vi "Settings.vi"(8 "Error In":errorcluster, 10 "Manual":path=path "", 11 "Settings in":T11={"MFIA"={"Address"="", "Use compensation"=TRUE, "Shut down gracefully"=FALSE}, "Temp ctrl"={"Gain (P)"=0.0, "Reset (I)"=0.0, "Rate (D)"=0.0, "Stabilization rate"=0.0, "Stabilization delta"=0.0, "Type"=enum."Lake Shore 325", "Custom temp ctrl"={"VISA resource name"=""}, "Lakeshore 325"={"VISA name"="", "Loop"=0, "Heater Range"=1, "Heater Resistance"=0, "Sample sensor"=0, "Fast sensor"=0, "Slow sensor"=0}, "Lakeshore 331"={"VISA name"="", "Loop"=1, "Heater Range"=0, "Sample sensor"=0, "Fast sensor"=0, "Slow sensor"=0}, "Lakeshore 332"={"VISA name"="", "Loop"=1, "Heater Range"=0, "Sample sensor"=0, "Fast sensor"=0, "Slow sensor"=0}, "Lakeshore 335"={"VISA name"="", "Loop"=1, "Sample sensor"=0, "Fast sensor"=0, "Slow sensor"=0, "Heater Range"=0, "Heater Output"=1, "Output mode"=enum."Off"}}, "Source-meter"={"Type"=enum."Custom", "Custom source-meter"={"VISA resource name"=""}, "Keithley 2600"={"VISA name"=""}}, "Other"={"Enable OriginLab"=FALSE, "Reader mode"=FALSE, "Auto-save"=FALSE}, "Defaults"={"IV properties"={"T"=0.0, "Vstart"=-0.5, "Vstop"=0.5, "Vpoints"=10.0, "Settling"=0.01, "I limit"=-3.0, "Log mapping"=FALSE, "Averaging"=0.0}, "CV properties"={"T"=0.0, "Vstart"=-0.5, "Vstop"=0.5, "Vpoints"=10.0, "Precision"=enum."Normal", "Test signal"=0.01, "Auto I range"=FALSE, "Test frequency"=100000.0, "I range"=-2.0, "V range"=10.0, "Log mapping"=FALSE, "Rel perm"=0.0, "Area"=0.0}, "DLTS properties"={"Tstart"=0.0, "Instant start"=FALSE, "Tstop"=0.0, "T rate"=0.0, "Test signal"=0.0, "Test frequency"=0.0, "Bandwidth"=0.0, "Averaging"=0.0, "Vbias"=0.0, "Vpulse"=0.0, "pulse length"=0.0, "Pulse 2"=FALSE, "Vpulse 2"=0.0, "pulse length 2"=0.0, "I range"=-2.0, "V range"=10.0, "Emission rate"=[], "Sampling rate"=0.0, "Acq. delay"=0.0}, "LDLTS properties"={"T"=0.0, "Test signal"=0.0, "Test frequency"=0.0, "Bandwidth"=0.0, "Averaging"=0.0, "Vbias"=0.0, "Vpulse"=0.0, "pulse length"=0.0, "Pulse 2"=FALSE, "Vpulse 2"=0.0, "pulse length 2"=0.0, "I range"=-2.0, "V range"=10.0, "Sampling rate"=0.0, "Acq. delay"=0.0, "Sampling time"=0.0}}} {"Defaults"."LDLTS properties"."V range" items=["10mV"=0.01, "100mV"=0.1, "1V"=1.0, "10V"=10.0]; "Defaults"."LDLTS properties"."I range" items=["100nA"=-7.0, "1µA"=-6.0, "10µA"=-5.0, "100µA"=-4.0, "1mA"=-3.0, "10mA"=-2.0]; "Defaults"."DLTS properties"."V range" items=["10mV"=0.01, "100mV"=0.1, "1V"=1.0, "10V"=10.0]; "Defaults"."DLTS properties"."I range" items=["10mV"=0.01, "100mV"=0.1, "1V"=1.0, "10V"=10.0]; "Defaults"."CV properties"."V range" items=["10mV"=0.01, "100mV"=0.1, "1V"=1.0, "10V"=10.0]; "Defaults"."CV properties"."I range" items=["100nA"=-7.0, "1µA"=-6.0, "10µA"=-5.0, "100µA"=-4.0, "1mA"=-3.0, "10mA"=-2.0]; "Defaults"."IV properties"."Settling" min=0.0 max=65535.0; "Temp ctrl"."Lakeshore 335"."Heater Output" items=["1"=1, "2"=2]; "Temp ctrl"."Lakeshore 335"."Heater Range" items=["Off", "Low (On)", "Medium", "High"]; "Temp ctrl"."Lakeshore 335"."Slow sensor" items=["A", "B"]; "Temp ctrl"."Lakeshore 335"."Fast sensor" items=["A", "B"]; "Temp ctrl"."Lakeshore 335"."Sample sensor" items=["A", "B"]; "Temp ctrl"."Lakeshore 335"."Loop" items=["Loop 1"=1, "Loop 2"=2]; "Temp ctrl"."Lakeshore 332"."Slow sensor" items=["A", "B"]; "Temp ctrl"."Lakeshore 332"."Fast sensor" items=["A", "B"]; "Temp ctrl"."Lakeshore 332"."Sample sensor" items=["A", "B"]; "Temp ctrl"."Lakeshore 332"."Heater Range" items=["Off", "Low (0.5W)", "Med (5W)", "High (50W)"]; "Temp ctrl"."Lakeshore 332"."Loop" items=["Loop 1", "Loop 2"]; "Temp ctrl"."Lakeshore 331"."Slow sensor" items=["A", "B"]; "Temp ctrl"."Lakeshore 331"."Fast sensor" items=["A", "B"]; "Temp ctrl"."Lakeshore 331"."Sample sensor" items=["A", "B"]; "Temp ctrl"."Lakeshore 331"."Heater Range" items=["Off", "Low (0.5W)", "Med (5W)", "High (50W)"]; "Temp ctrl"."Lakeshore 331"."Loop" items=["Loop 1", "Loop 2"]; "Temp ctrl"."Lakeshore 325"."Slow sensor" items=["A", "B"]; "Temp ctrl"."Lakeshore 325"."Fast sensor" items=["A", "B"]; "Temp ctrl"."Lakeshore 325"."Sample sensor" items=["A", "B"]; "Temp ctrl"."Lakeshore 325"."Heater Resistance" items=["25 Ohm"=1, "50 Ohm"=2]; "Temp ctrl"."Lakeshore 325"."Heater Range" items=["Off", "Low (loop 1) or On (loop 2)", "High (loop 1)"]; "Temp ctrl"."Lakeshore 325"."Loop" items=["Loop 1"=1, "Loop 2"=2]}) -> (0 "Error Out":errorcluster, 3 "Settings":T11={"MFIA"={"Address"="", "Use compensation"=TRUE, "Shut down gracefully"=FALSE}, "Temp ctrl"={"Gain (P)"=0.0, "Reset (I)"=0.0, "Rate (D)"=0.0, "Stabilization rate"=0.0, "Stabilization delta"=0.0, "Type"=enum."Lake Shore 325", "Custom temp ctrl"={"VISA resource name"=""}, "Lakeshore 325"={"VISA name"="", "Loop"=0, "Heater Range"=1, "Heater Resistance"=0, "Sample sensor"=0, "Fast sensor"=0, "Slow sensor"=0}, "Lakeshore 331"={"VISA name"="", "Loop"=1, "Heater Range"=0, "Sample sensor"=0, "Fast sensor"=0, "Slow sensor"=0}, "Lakeshore 332"={"VISA name"="", "Loop"=1, "Heater Range"=0, "Sample sensor"=0, "Fast sensor"=0, "Slow sensor"=0}, "Lakeshore 335"={"VISA name"="", "Loop"=1, "Sample sensor"=0, "Fast sensor"=0, "Slow sensor"=0, "Heater Range"=0, "Heater Output"=1, "Output mode"=enum."Off"}}, "Source-meter"={"Type"=enum."Custom", "Custom source-meter"={"VISA resource name"=""}, "Keithley 2600"={"VISA name"=""}}, "Other"={"Enable OriginLab"=FALSE, "Reader mode"=FALSE, "Auto-save"=FALSE}, "Defaults"={"IV properties"={"T"=0.0, "Vstart"=-0.5, "Vstop"=0.5, "Vpoints"=10.0, "Settling"=0.01, "I limit"=-3.0, "Log mapping"=FALSE, "Averaging"=0.0}, "CV properties"={"T"=0.0, "Vstart"=-0.5, "Vstop"=0.5, "Vpoints"=10.0, "Precision"=enum."Normal", "Test signal"=0.01, "Auto I range"=FALSE, "Test frequency"=100000.0, "I range"=-2.0, "V range"=10.0, "Log mapping"=FALSE, "Rel perm"=0.0, "Area"=0.0}, "DLTS properties"={"Tstart"=0.0, "Instant start"=FALSE, "Tstop"=0.0, "T rate"=0.0, "Test signal"=0.0, "Test frequency"=0.0, "Bandwidth"=0.0, "Averaging"=0.0, "Vbias"=0.0, "Vpulse"=0.0, "pulse length"=0.0, "Pulse 2"=FALSE, "Vpulse 2"=0.0, "pulse length 2"=0.0, "I range"=-2.0, "V range"=10.0, "Emission rate"=[], "Sampling rate"=0.0, "Acq. delay"=0.0}, "LDLTS properties"={"T"=0.0, "Test signal"=0.0, "Test frequency"=0.0, "Bandwidth"=0.0, "Averaging"=0.0, "Vbias"=0.0, "Vpulse"=0.0, "pulse length"=0.0, "Pulse 2"=FALSE, "Vpulse 2"=0.0, "pulse length 2"=0.0, "I range"=-2.0, "V range"=10.0, "Sampling rate"=0.0, "Acq. delay"=0.0, "Sampling time"=0.0}}} {"Defaults"."LDLTS properties"."V range" items=["10mV"=0.01, "100mV"=0.1, "1V"=1.0, "10V"=10.0]; "Defaults"."LDLTS properties"."I range" items=["100nA"=-7.0, "1µA"=-6.0, "10µA"=-5.0, "100µA"=-4.0, "1mA"=-3.0, "10mA"=-2.0]; "Defaults"."DLTS properties"."V range" items=["10mV"=0.01, "100mV"=0.1, "1V"=1.0, "10V"=10.0]; "Defaults"."DLTS properties"."I range" items=["10mV"=0.01, "100mV"=0.1, "1V"=1.0, "10V"=10.0]; "Defaults"."CV properties"."V range" items=["10mV"=0.01, "100mV"=0.1, "1V"=1.0, "10V"=10.0]; "Defaults"."CV properties"."I range" items=["100nA"=-7.0, "1µA"=-6.0, "10µA"=-5.0, "100µA"=-4.0, "1mA"=-3.0, "10mA"=-2.0]; "Defaults"."IV properties"."Settling" min=0.0 max=65535.0; "Temp ctrl"."Lakeshore 335"."Heater Output" items=["1"=1, "2"=2]; "Temp ctrl"."Lakeshore 335"."Heater Range" items=["Off", "Low (On)", "Medium", "High"]; "Temp ctrl"."Lakeshore 335"."Slow sensor" items=["A", "B"]; "Temp ctrl"."Lakeshore 335"."Fast sensor" items=["A", "B"]; "Temp ctrl"."Lakeshore 335"."Sample sensor" items=["A", "B"]; "Temp ctrl"."Lakeshore 335"."Loop" items=["Loop 1"=1, "Loop 2"=2]; "Temp ctrl"."Lakeshore 332"."Slow sensor" items=["A", "B"]; "Temp ctrl"."Lakeshore 332"."Fast sensor" items=["A", "B"]; "Temp ctrl"."Lakeshore 332"."Sample sensor" items=["A", "B"]; "Temp ctrl"."Lakeshore 332"."Heater Range" items=["Off", "Low (0.5W)", "Med (5W)", "High (50W)"]; "Temp ctrl"."Lakeshore 332"."Loop" items=["Loop 1", "Loop 2"]; "Temp ctrl"."Lakeshore 331"."Slow sensor" items=["A", "B"]; "Temp ctrl"."Lakeshore 331"."Fast sensor" items=["A", "B"]; "Temp ctrl"."Lakeshore 331"."Sample sensor" items=["A", "B"]; "Temp ctrl"."Lakeshore 331"."Heater Range" items=["Off", "Low (0.5W)", "Med (5W)", "High (50W)"]; "Temp ctrl"."Lakeshore 331"."Loop" items=["Loop 1", "Loop 2"]; "Temp ctrl"."Lakeshore 325"."Slow sensor" items=["A", "B"]; "Temp ctrl"."Lakeshore 325"."Fast sensor" items=["A", "B"]; "Temp ctrl"."Lakeshore 325"."Sample sensor" items=["A", "B"]; "Temp ctrl"."Lakeshore 325"."Heater Resistance" items=["25 Ohm"=1, "50 Ohm"=2]; "Temp ctrl"."Lakeshore 325"."Heater Range" items=["Off", "Low (loop 1) or On (loop 2)", "High (loop 1)"]; "Temp ctrl"."Lakeshore 325"."Loop" items=["Loop 1"=1, "Loop 2"=2]})   [LabVIEW 2019]
doc: "Displays a window that enabling user to modify the settings"
uses:
  Type defs/Settings Type Def.ctl
  Type defs/Imps Type Def.ctl
  Type defs/Temp ctrl Type Def.ctl
  Custom devices/Custom temp ctrl settings.ctl
  Type defs/Source-meter Type Def.ctl
  Custom devices/Custom source-meter settings.ctl
  Type defs/Other settings Type Def.ctl
  Type defs/IV properties Type Def.ctl
  Type defs/CV properties Type Def.ctl
  Type defs/DLTS properties Type Def.ctl
  Type defs/LDLTS properties Type Def.ctl
  <vilib>/Utility/miscctls.llb/LVPointTypeDef.ctl
  <instrlib>/Zurich Instruments LabOne/Zurich Instruments LabOne.lvlib
panel:
  in  "Help":bool
  in  "Tab Control":T1(tab)
  in  "Address":string(combo) caption="Combo Box"
  in  "Refresh":bool
  in  "Use user compensation":bool
  in  "Safely shutdown on exit":bool
  in  "Stabilization delta":dbl[unit] caption="Numeric"
  in  "Stabilization rate":dbl[unit] caption="Numeric"
  in  "Temp type":T2(tab)
  in  "Custom temp ctrl":T3
  in  "Fast sensor LS325":u16(ring)=1 caption="Fast sensor" items=["Sensor A", "Sensor B"]
  in  "Slow sensor LS325":u16(ring)=1 caption="Slow sensor" items=["Sensor A", "Sensor B"]
  in  "Sample sensor LS325":u16(ring)=1 caption="Sample sensor" items=["Sensor A", "Sensor B"]
  in  "Heater range LS325":u16(ring)=1 caption="Heater range" items=["Off", "Low (L1)/On (L2)", "High (L1)"]
  in  "Loop  LS325":u16(ring)=1 caption="Loop" items=["Loop 1"=1, "Loop 2"=2]
  in  "VISA name LS325":refnum<visa-resource-name> caption="VISA name"
  in  "Heater resistance LS325":u16(ring)=1 caption="Heater resistance" items=["25 Ohm"=1, "50 Ohm"=2]
  in  "Fast sensor LS331":u16(ring)=1 caption="Fast sensor" items=["Sensor A", "Sensor B"]
  in  "Slow sensor LS331":u16(ring)=1 caption="Slow sensor" items=["Sensor A", "Sensor B"]
  in  "Sample sensor LS331":u16(ring)=1 caption="Sample sensor" items=["Sensor A", "Sensor B"]
  in  "Heater range LS331":u16(ring)=1 caption="Heater range" items=["Off", "Low (0.5W)", "Med (5W)", "High (50W)"]
  in  "Loop  LS331":u16(ring)=1 caption="Loop" items=["Loop 1", "Loop 2"]
  in  "VISA name LS331":refnum<visa-resource-name> caption="VISA name"
  in  "Fast sensor LS332":u16(ring)=1 caption="Fast sensor" items=["Sensor A", "Sensor B"]
  in  "Slow sensor LS332":u16(ring)=1 caption="Slow sensor" items=["Sensor A", "Sensor B"]
  in  "Sample sensor LS332":u16(ring)=1 caption="Sample sensor" items=["Sensor A", "Sensor B"]
  in  "Heater range LS332":u16(ring)=1 caption="Heater range" items=["Off", "Low (0.5W)", "Med (5W)", "High (50W)"]
  in  "Loop  LS332":u16(ring)=1 caption="Loop" items=["Loop 1", "Loop 2"]
  in  "VISA name LS332":refnum<visa-resource-name> caption="VISA name"
  in  "Heater range LS335":enum16{"Off", "Low/On", "Medium", "High"}(ring) caption="Heater range"
  in  "Output mode LS335":T4(ring) caption="Output mode"
  in  "Heater output LS335":u16=1 caption="Heater output" min=1 max=2 step=1
  in  "Fast sensor LS335":u16(ring)=1 caption="Fast sensor" items=["Sensor A", "Sensor B"]
  in  "Slow sensor LS335":u16(ring)=1 caption="Slow sensor" items=["Sensor A", "Sensor B"]
  in  "Sample sensor LS335":u16(ring)=1 caption="Sample sensor" items=["Sensor A", "Sensor B"]
  in  "Loop  LS335":u16(ring)=1 caption="Loop" items=["Loop 1"=1, "Loop 2"=2]
  in  "VISA name LS335":refnum<visa-resource-name> caption="VISA name"
  in  "PID":T5
  in  "Source-meter type":enum32{"Custom", "Keithley 2600"}(tab)
  in  "Custom source-meter":T6
  in  "VISA name Keithley 2600":refnum<visa-resource-name> caption="VISA name"
  in  "Defaults tab control":enum32{"CV", "IV", "DLTS", "LDLTS"}(tab)
  in  "CV properties":T7={"T"=0.0, "Vstart"=-0.5, "Vstop"=0.5, "Vpoints"=10.0, "Precision"=enum."Normal", "Test signal"=0.01, "Auto I range"=FALSE, "Test frequency"=100000.0, "I range"=-2.0, "V range"=10.0, "Log mapping"=FALSE, "Rel perm"=0.0, "Area"=0.0} {"V range" items=["10mV"=0.01, "100mV"=0.1, "1V"=1.0, "10V"=10.0]; "I range" items=["100nA"=-7.0, "1µA"=-6.0, "10µA"=-5.0, "100µA"=-4.0, "1mA"=-3.0, "10mA"=-2.0]}
  in  "IV properties":T8={"T"=0.0, "Vstart"=-0.5, "Vstop"=0.5, "Vpoints"=10.0, "Settling"=0.01, "I limit"=-3.0, "Log mapping"=FALSE, "Averaging"=0.0} {"Settling" min=0.0 max=65535.0}
  in  "DLTS properties":T9={"Tstart"=0.0, "Instant start"=FALSE, "Tstop"=0.0, "T rate"=0.0, "Test signal"=0.0, "Test frequency"=0.0, "Bandwidth"=0.0, "Averaging"=0.0, "Vbias"=0.0, "Vpulse"=0.0, "pulse length"=0.0, "Pulse 2"=FALSE, "Vpulse 2"=0.0, "pulse length 2"=0.0, "I range"=-2.0, "V range"=10.0, "Emission rate"=[], "Sampling rate"=0.0, "Acq. delay"=0.0} {"Sampling rate" items=["13k"=13392.857422, "27k"=26785.714844, "54k"=53571.429687, "107k"=107142.859375]; "V range" items=["10mV"=0.01, "100mV"=0.1, "1V"=1.0, "10V"=10.0]; "I range" items=["100nA"=-7.0, "1µA"=-6.0, "10µA"=-5.0, "100µA"=-4.0, "1mA"=-3.0, "10mA"=-2.0]}
  in  "LDLTS properties":T10={"T"=0.0, "Test signal"=0.0, "Test frequency"=0.0, "Bandwidth"=0.0, "Averaging"=0.0, "Vbias"=0.0, "Vpulse"=0.0, "pulse length"=0.0, "Pulse 2"=FALSE, "Vpulse 2"=0.0, "pulse length 2"=0.0, "I range"=-2.0, "V range"=10.0, "Sampling rate"=0.0, "Acq. delay"=0.0, "Sampling time"=0.0} {"Sampling rate" items=["13k"=13392.857422, "27k"=26785.714844, "54k"=53571.429687, "107k"=107142.859375]; "V range" items=["10mV"=0.01, "100mV"=0.1, "1V"=1.0, "10V"=10.0]; "I range" items=["100nA"=-7.0, "1µA"=-6.0, "10µA"=-5.0, "100µA"=-4.0, "1mA"=-3.0, "10mA"=-2.0]}
  in  "Reader mode":bool
  in  "Enable Origin":bool caption="Enable OriginLab"
  in  "Auto-save":bool
  in  "Cancel":bool
  in  "Apply All":bool
  # "Warning! This device has not been tested with myDLTS"
  # "Warning! This device has not been tested with myDLTS"
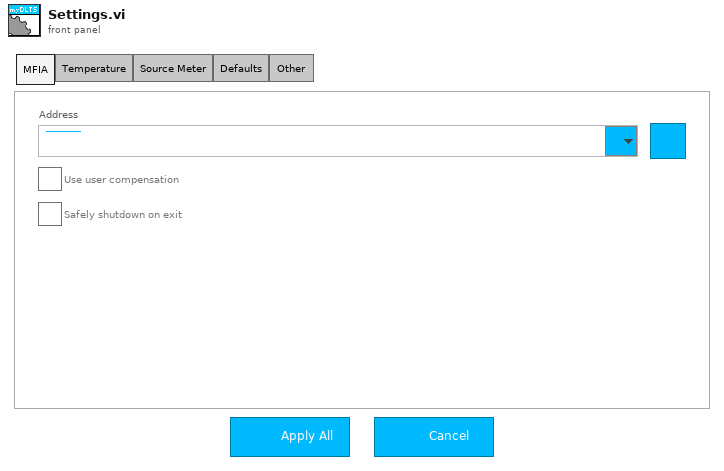
[diagram p1: front panel]
types:
  T1 = enum32{"MFIA", "Temperature", "Source Meter", "Defaults", "Other "}
  T2 = enum32{"Custom", "Lake Shore 325", "Lake Shore 331", "Lake Shore 332", "Lake Shore 335"}
  T3 = typedef "Custom temp ctrl settings.ctl" = cluster{"VISA resource name":refnum<visa-resource-name>}
  T4 = enum16{"Off", "Closed Loop PID", "Zone", "Open Loop", "Monitor Out", "Warmup Supply"}
  T5 = cluster{"Gain (P)":dbl, "Reset (I)":dbl, "Rate (D)":u16}
  T6 = typedef "Custom source-meter settings.ctl" = cluster{"VISA resource name":refnum<visa-resource-name>}
  T7 = typedef "CV properties Type Def.ctl" = cluster{"T":dbl[unit], "Vstart":dbl[unit], "Vstop":dbl[unit], "Vpoints":dbl, "Precision":enum16{"Low (Fast)", "Normal", "High (Slow)"}, "Test signal":dbl[unit], "Auto I range":bool, "Test frequency":dbl[unit], "I range":dbl, "V range":dbl[unit], "Log mapping":bool, "Rel perm":dbl, "Area":dbl[unit]}
  T8 = typedef "IV properties Type Def.ctl" = cluster{"T":dbl[unit], "Vstart":dbl[unit], "Vstop":dbl[unit], "Vpoints":dbl, "Settling":dbl[unit], "I limit":dbl[unit], "Log mapping":bool, "Averaging":dbl}
  T9 = typedef "DLTS properties Type Def.ctl" = cluster{"Tstart":dbl[unit], "Instant start":bool, "Tstop":dbl[unit], "T rate":dbl[unit], "Test signal":dbl[unit], "Test frequency":dbl[unit], "Bandwidth":dbl[unit], "Averaging":dbl, "Vbias":dbl[unit], "Vpulse":dbl[unit], "pulse length":dbl[unit], "Pulse 2":bool, "Vpulse 2":dbl[unit], "pulse length 2":dbl[unit], "I range":dbl, "V range":dbl[unit], "Emission rate":dbl[unit][], "Sampling rate":dbl[unit], "Acq. delay":dbl[unit]}
  T10 = typedef "LDLTS properties Type Def.ctl" = cluster{"T":dbl[unit], "Test signal":dbl[unit], "Test frequency":dbl[unit], "Bandwidth":dbl[unit], "Averaging":dbl, "Vbias":dbl[unit], "Vpulse":dbl[unit], "pulse length":dbl[unit], "Pulse 2":bool, "Vpulse 2":dbl[unit], "pulse length 2":dbl[unit], "I range":dbl, "V range":dbl[unit], "Sampling rate":dbl[unit], "Acq. delay":dbl[unit], "Sampling time":dbl[unit]}
  T11 = typedef "Settings Type Def.ctl" = cluster{"MFIA":T12, "Temp ctrl":T13, "Source-meter":T14, "Other":T15, "Defaults":cluster{"IV properties":T8, "CV properties":T7, "DLTS properties":T9, "LDLTS properties":T10}}
  T12 = typedef "Imps Type Def.ctl" = cluster{"Address":string, "Use compensation":bool, "Shut down gracefully":bool}
  T13 = typedef "Temp ctrl Type Def.ctl" = cluster{"Gain (P)":dbl, "Reset (I)":dbl, "Rate (D)":dbl, "Stabilization rate":dbl, "Stabilization delta":dbl, "Type":enum16{"Custom", "Lake Shore 325", "Lake Shore 331", "Lake Shore 332", "Lake Shore 335"}, "Custom temp ctrl":T3, "Lakeshore 325":cluster{"VISA name":refnum<visa-resource-name>, "Loop":u16, "Heater Range":u16, "Heater Resistance":u16, "Sample sensor":u16, "Fast sensor":u16, "Slow sensor":u16}, "Lakeshore 331":cluster{"VISA name":refnum<visa-resource-name>, "Loop":u16, "Heater Range":u16, "Sample sensor":u16, "Fast sensor":u16, "Slow sensor":u16}, "Lakeshore 332":cluster{"VISA name":refnum<visa-resource-name>, "Loop":u16, "Heater Range":u16, "Sample sensor":u16, "Fast sensor":u16, "Slow sensor":u16}, "Lakeshore 335":cluster{"VISA name":refnum<visa-resource-name>, "Loop":u16, "Sample sensor":u16, "Fast sensor":u16, "Slow sensor":u16, "Heater Range":u16, "Heater Output":u16, "Output mode":enum16{"Off", "Closed Loop PID", "Zone", "Open Loop", "Monitor Out", "Warmup Supply"}}}
  T14 = typedef "Source-meter Type Def.ctl" = cluster{"Type":enum16{"Custom", "Keithley 2600"}, "Custom source-meter":T6, "Keithley 2600":cluster{"VISA name":refnum<visa-resource-name>}}
  T15 = typedef "Other settings Type Def.ctl" = cluster{"Enable OriginLab":bool, "Reader mode":bool, "Auto-save":bool}
  T16 = typedef "LVPointTypeDef.ctl" = cluster{"Horizontal":i16, "Vertical":i16}
  T17 = enum16{"Custom", "Lake Shore 325", "Lake Shore 331", "Lake Shore 332", "Lake Shore 335"}
  T18 = cluster{"Rate (D)":dbl, "Reset (I)":dbl, "Gain (P)":dbl}
  T19 = enum8{"Enabled", "Disabled", "Disabled and Grayed Out"}
  T20 = cluster{"VISA name LS335":refnum<visa-resource-name>, "Loop  LS335":u16, "Sample sensor LS335":u16, "Fast sensor LS335":u16, "Slow sensor LS335":u16, "Heater range LS335":enum16{"Off", "Low/On", "Medium", "High"}, "Heater output LS335":u16, "Output mode LS335":enum16{"Off", "Closed Loop PID", "Zone", "Open Loop", "Monitor Out", "Warmup Supply"}}
  T21 = cluster{"VISA name LS332":refnum<visa-resource-name>, "Loop  LS332":u16, "Heater range LS332":u16, "Sample sensor LS332":u16, "Fast sensor LS332":u16, "Slow sensor LS332":u16}
  T22 = cluster{"VISA name LS331":refnum<visa-resource-name>, "Loop  LS331":u16, "Heater range LS331":u16, "Sample sensor LS331":u16, "Fast sensor LS331":u16, "Slow sensor LS331":u16}
  T23 = typedef "Zurich Instruments LabOne.lvlib/ziTypeHandle.ctl" = cluster{"handleValid":bool, "Conn":u64, "Path Prefix":string, "Handle":u64, "Connected":bool, "Clockbase(s)":dbl}
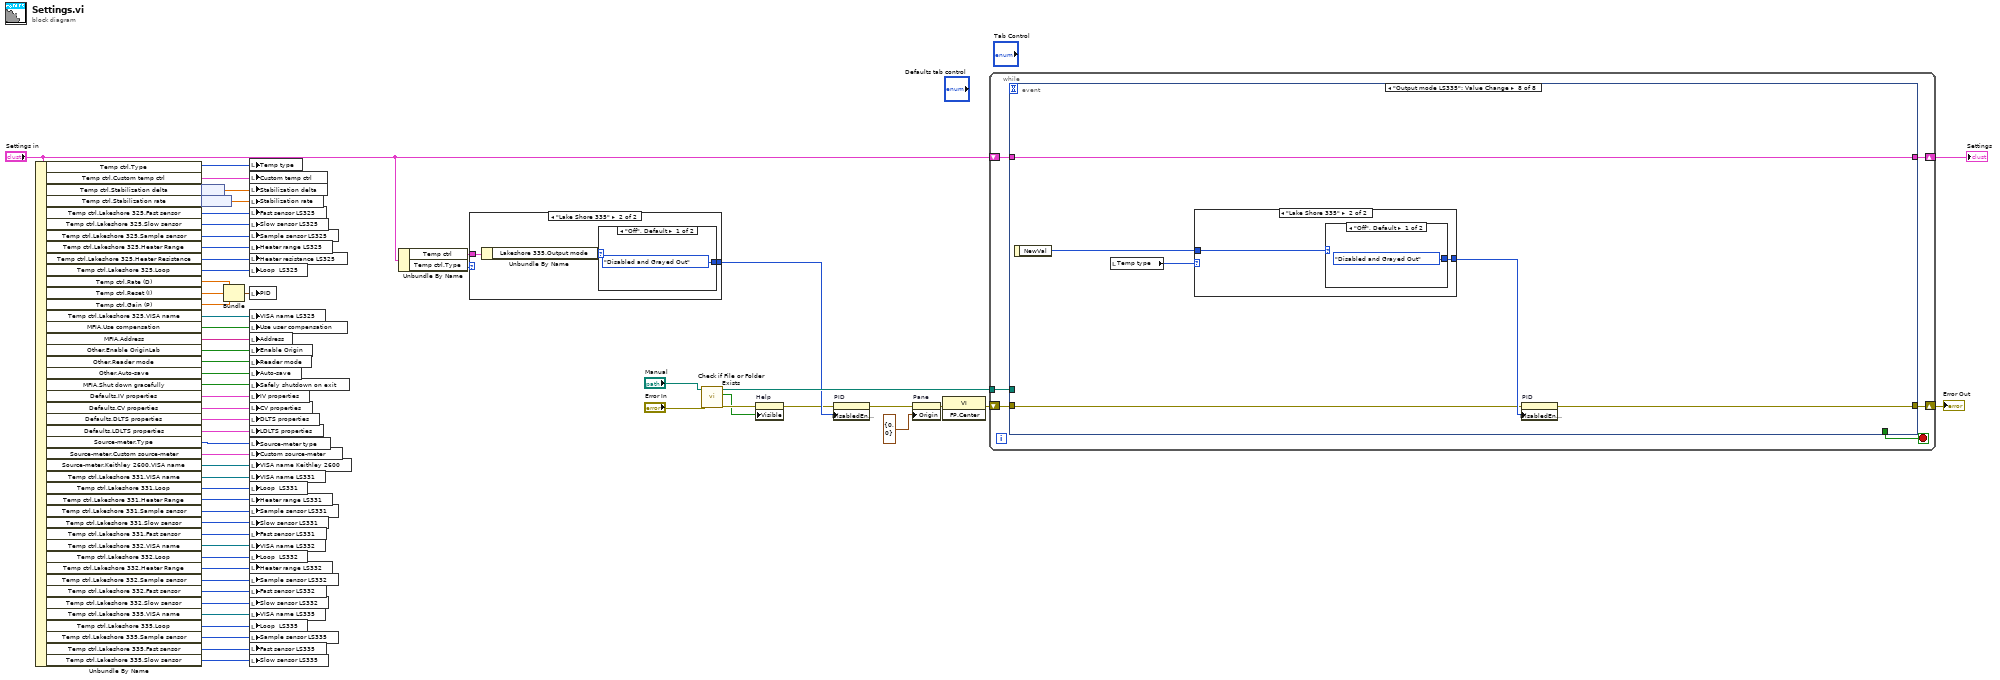
[diagram p0: block diagram]
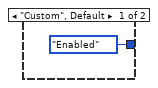
[diagram p2: hidden frame]
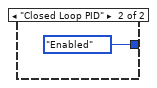
[diagram p3: hidden frame]
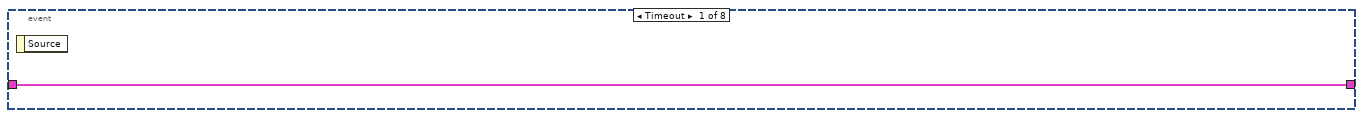
[diagram p4: hidden frame]
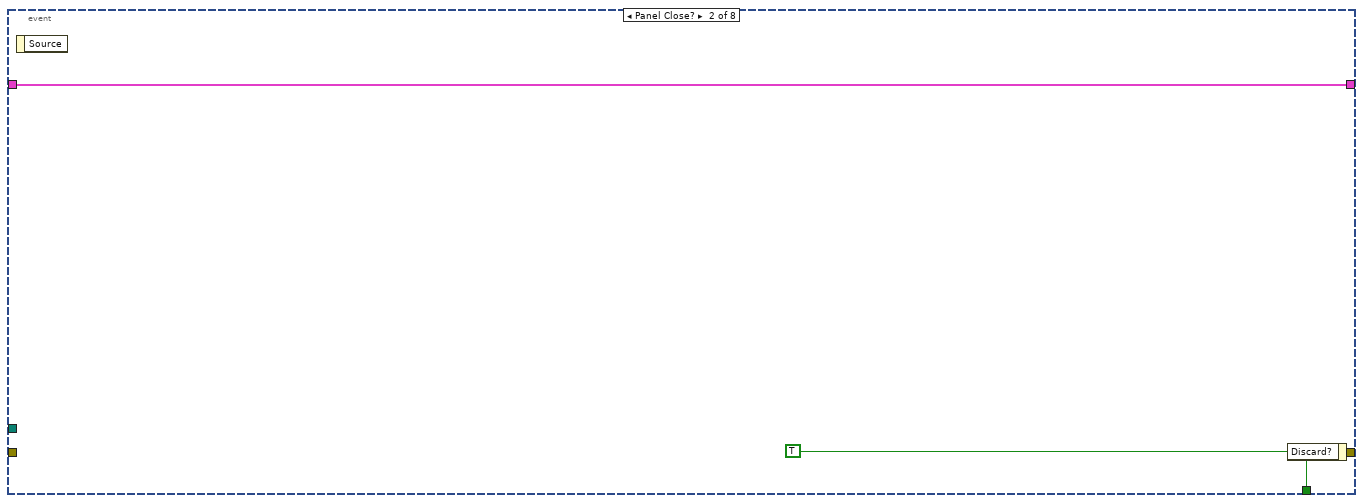
[diagram p5: hidden frame]
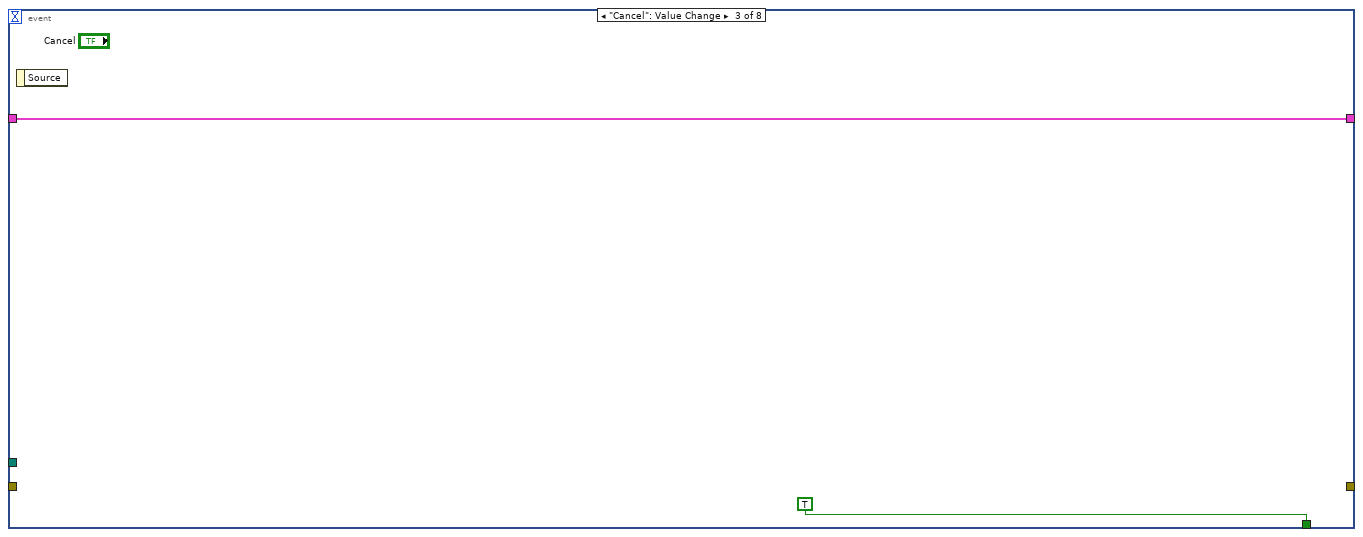
[diagram p6: hidden frame]
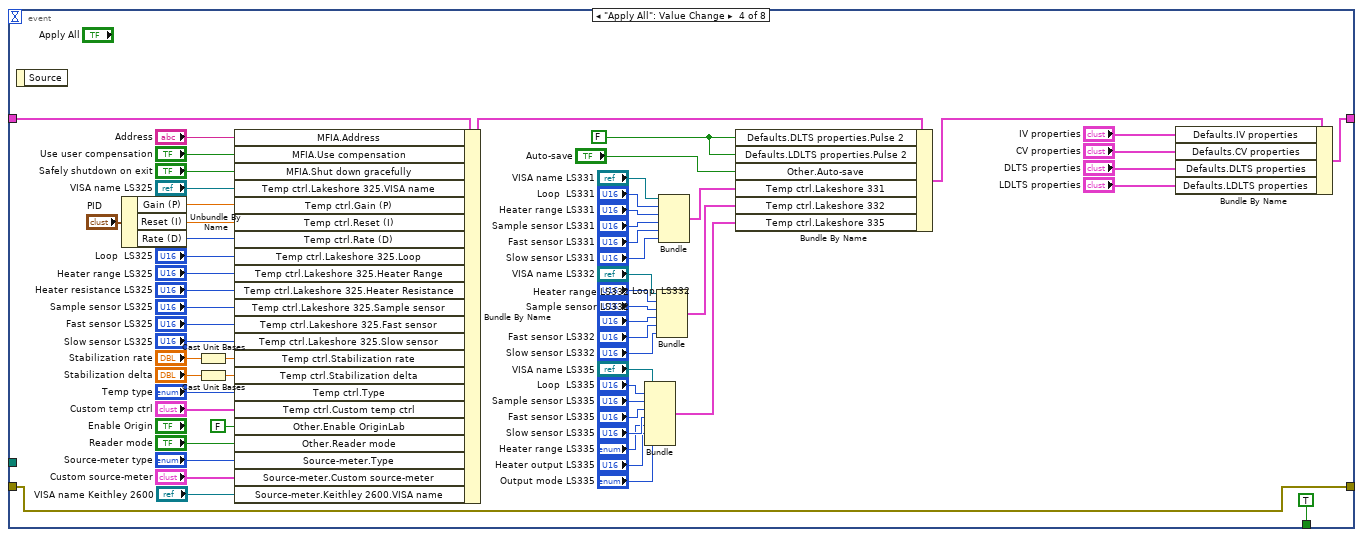
[diagram p7: hidden frame]
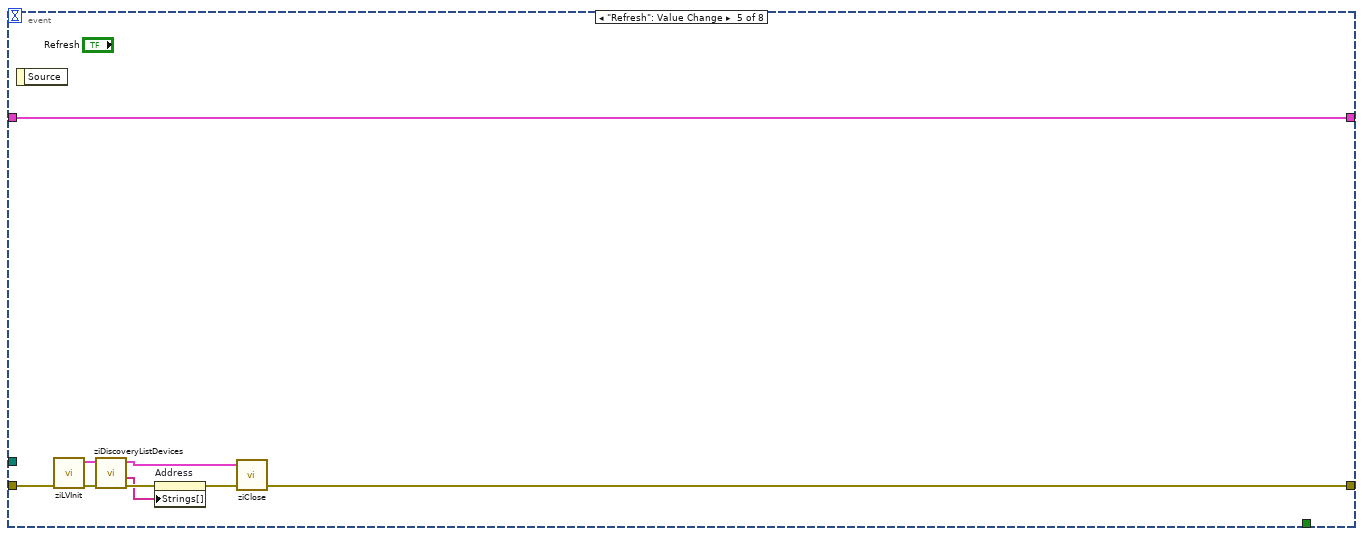
[diagram p8: hidden frame]
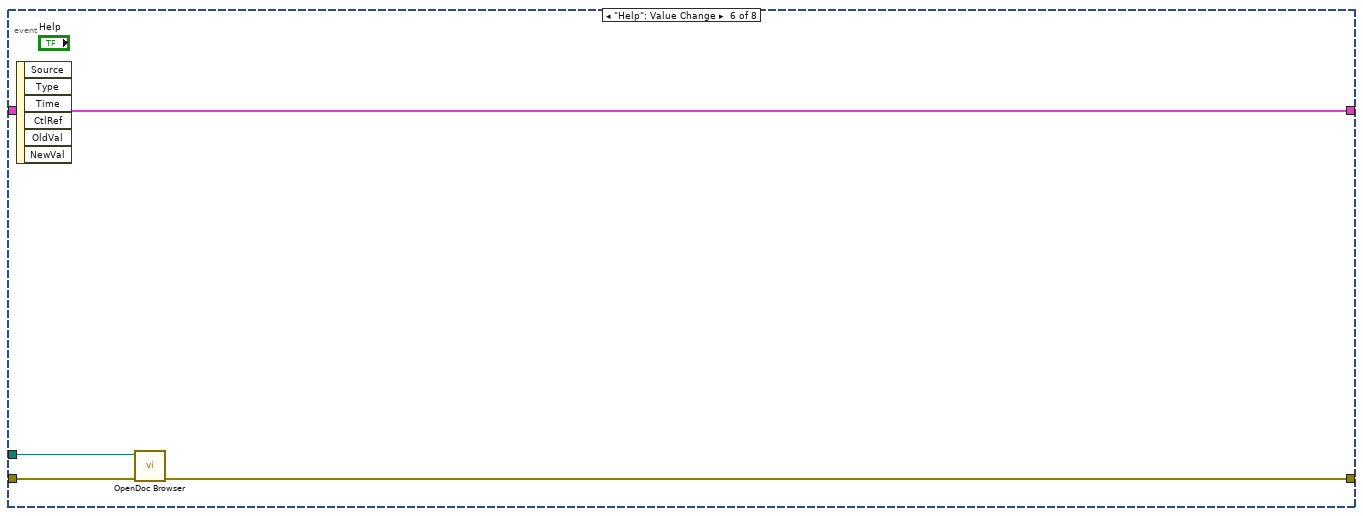
[diagram p9: hidden frame]
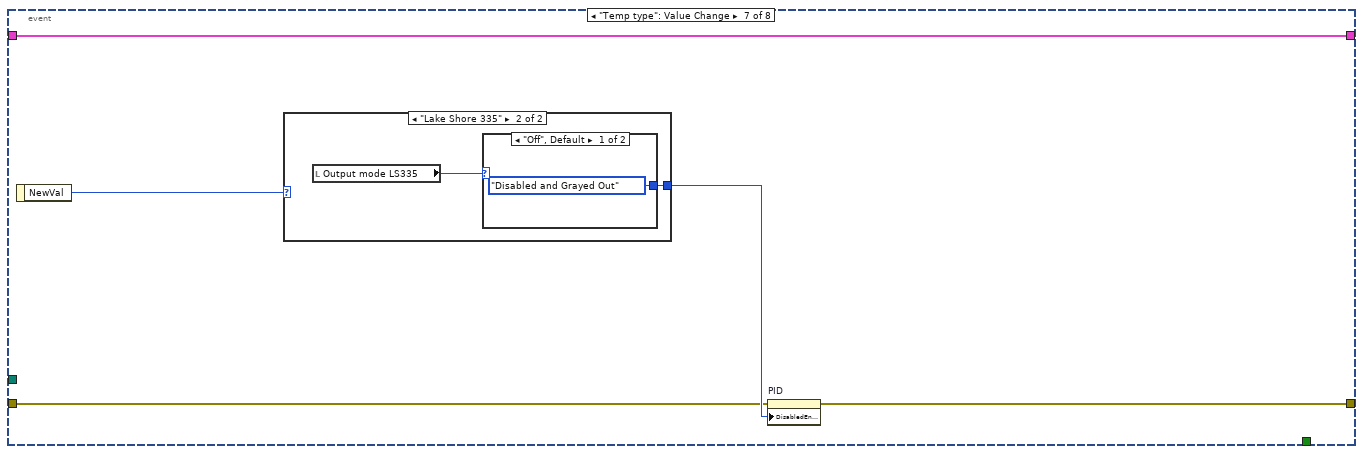
[diagram p10: hidden frame]
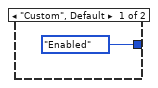
[diagram p11: hidden frame]
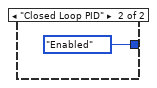
[diagram p12: hidden frame]
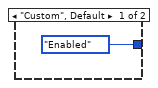
[diagram p13: hidden frame]
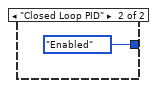
[diagram p14: hidden frame]
diagram:
  n1 = Unbundle By Name("Settings in") -> ("Temp ctrl.Type"=w37:T17, "Temp ctrl.Custom temp ctrl"=w38:T3, "Temp ctrl.Stabilization delta"=w63:dbl, "Temp ctrl.Stabilization rate"=w62:dbl, "Temp ctrl.Lakeshore 325.Fast sensor"=w61:u16, "Temp ctrl.Lakeshore 325.Slow sensor"=w60:u16, "Temp ctrl.Lakeshore 325.Sample sensor"=w59:u16, "Temp ctrl.Lakeshore 325.Heater Range"=w58:u16, "Temp ctrl.Lakeshore 325.Heater Resistance"=w57:u16, "Temp ctrl.Lakeshore 325.Loop"=w56:u16, "Temp ctrl.Rate (D)"=w10:dbl, "Temp ctrl.Reset (I)"=w9:dbl, "Temp ctrl.Gain (P)"=w8:dbl, "Temp ctrl.Lakeshore 325.VISA name"=w53:refnum<visa-resource-name>, "MFIA.Use compensation"=w54:bool, "MFIA.Address"=w55:string, "Other.Enable OriginLab"=w49:bool, "Other.Reader mode"=w36:bool, "Other.Auto-save"=w11:bool, "MFIA.Shut down gracefully"=w44:bool, "Defaults.IV properties"=w35:T8, "Defaults.CV properties"=w34:T7, "Defaults.DLTS properties"=w33:T9, "Defaults.LDLTS properties"=w32:T10, "Source-meter.Type"=w30:enum16{"Custom", "Keithley 2600"}, "Source-meter.Custom source-meter"=w29:T6, "Source-meter.Keithley 2600.VISA name"=w31:refnum<visa-resource-name>, "Temp ctrl.Lakeshore 331.VISA name"=w28:refnum<visa-resource-name>, "Temp ctrl.Lakeshore 331.Loop"=w27:u16, "Temp ctrl.Lakeshore 331.Heater Range"=w26:u16, "Temp ctrl.Lakeshore 331.Sample sensor"=w25:u16, "Temp ctrl.Lakeshore 331.Slow sensor"=w24:u16, "Temp ctrl.Lakeshore 331.Fast sensor"=w23:u16, "Temp ctrl.Lakeshore 332.VISA name"=w22:refnum<visa-resource-name>, "Temp ctrl.Lakeshore 332.Loop"=w21:u16, "Temp ctrl.Lakeshore 332.Heater Range"=w20:u16, "Temp ctrl.Lakeshore 332.Sample sensor"=w19:u16, "Temp ctrl.Lakeshore 332.Fast sensor"=w18:u16, "Temp ctrl.Lakeshore 332.Slow sensor"=w17:u16, "Temp ctrl.Lakeshore 335.VISA name"=w16:refnum<visa-resource-name>, "Temp ctrl.Lakeshore 335.Loop"=w15:u16, "Temp ctrl.Lakeshore 335.Sample sensor"=w14:u16, "Temp ctrl.Lakeshore 335.Fast sensor"=w13:u16, "Temp ctrl.Lakeshore 335.Slow sensor"=w12:u16)
  n2 = node(w63) -> (w48:dbl[unit])
  n3 = node(w62) -> (w47:dbl[unit])
  n4 = Bundle("Rate (D)"=w10, "Reset (I)"=w9, "Gain (P)"=w8) -> (w7:T18)  [unwired: 1 in]
  n5 = local write "Temp type"(w37) -> ()
  n6 = local write "Custom temp ctrl"(w38) -> ()
  n7 = local write "Stabilization delta"(w48) -> ()
  n8 = local write "Stabilization rate"(w47) -> ()
  n9 = local write "Fast sensor LS325"(w61) -> ()
  n10 = local write "Slow sensor LS325"(w60) -> ()
  n11 = local write "Sample sensor LS325"(w59) -> ()
  n12 = local write "Heater range LS325"(w58) -> ()
  n13 = local write "Heater resistance LS325"(w57) -> ()
  n14 = local write "Loop  LS325"(w56) -> ()
  n15 = local write "PID"(w7) -> ()
  n16 = local write "VISA name LS325"(w53) -> ()
  n17 = local write "Use user compensation"(w54) -> ()
  n18 = local write "Address"(w55) -> ()
  n19 = local write "Enable Origin"(w49) -> ()
  n20 = local write "Reader mode"(w36) -> ()
  n21 = local write "Auto-save"(w11) -> ()
  n22 = local write "Safely shutdown on exit"(w44) -> ()
  n23 = local write "IV properties"(w35) -> ()
  n24 = local write "CV properties"(w34) -> ()
  n25 = local write "DLTS properties"(w33) -> ()
  n26 = local write "LDLTS properties"(w32) -> ()
  n27 = local write "Source-meter type"(w30) -> ()
  n28 = local write "Custom source-meter"(w29) -> ()
  n29 = local write "VISA name Keithley 2600"(w31) -> ()
  n30 = local write "VISA name LS331"(w28) -> ()
  n31 = local write "Loop  LS331"(w27) -> ()
  n32 = local write "Heater range LS331"(w26) -> ()
  n33 = local write "Sample sensor LS331"(w25) -> ()
  n34 = local write "Slow sensor LS331"(w24) -> ()
  n35 = local write "Fast sensor LS331"(w23) -> ()
  n36 = local write "VISA name LS332"(w22) -> ()
  n37 = local write "Loop  LS332"(w21) -> ()
  n38 = local write "Heater range LS332"(w20) -> ()
  n39 = local write "Sample sensor LS332"(w19) -> ()
  n40 = local write "Fast sensor LS332"(w18) -> ()
  n41 = local write "Slow sensor LS332"(w17) -> ()
  n42 = local write "VISA name LS335"(w16) -> ()
  n43 = local write "Loop  LS335"(w15) -> ()
  n44 = local write "Sample sensor LS335"(w14) -> ()
  n45 = local write "Fast sensor LS335"(w13) -> ()
  n46 = local write "Slow sensor LS335"(w12) -> ()
  n47 = Unbundle By Name("Settings in") -> ("Temp ctrl"=w4:T13, "Temp ctrl.Type"=w5:T17)
  n48 = case shown="\"Lake Shore 335\"" w5 {
    tunnel: w4 -> [_ w67]
    tunnel: [T19."Enabled" ("Disabled") w65] -> w3
    frame "Custom", Default {
    }
    frame "Lake Shore 335" {
      n49 = Unbundle By Name(w67) -> ("Lakeshore 335.Output mode"=w66:T4)
      n50 = case shown="\"Off\", Default" w66 {
        tunnel: [T19."Disabled and Grayed Out" ("Disabled") T19."Enabled" ("Disabled")] -> w65
        frame "Off", Default {
        }
        frame "Closed Loop PID" {
        }
      }
    }
  }
  n51 = call <vilib>:"Check if File or Folder Exists.vi"("error in (no error)"="Error In", "path"="Manual") -> ("error out"=w40:errorcluster, "file or folder exists?"=w39:bool, "dup path"=w43:path)  [unwired: 7 in]
  n52 = property on="Help" class="Bool"(error in=w40, "Visible"=w39) -> (error out=w2:errorcluster)  [unwired: 1 in, 1 out]
  n53 = property on="PID" class="Clust (strict)"(error in=w2, "DisabledEnum"=w3) -> (error out=w1:errorcluster)  [unwired: 1 in, 1 out]
  n54 = property on="Pane" class="Pane"(error in=w1, "Origin"=T16 {"Horizontal"=0, "Vertical"=0}) -> (error out=w46:errorcluster)  [unwired: 1 in, 1 out]
  n55 = invoke class="VI" method="FP.Center"(error in=w46) -> (error out=w45:errorcluster)  [unwired: 2 in, 2 out]
  n56 = while {
    shift-right: [w73] -> w51
    shift-left: "Settings in" -> [w74]
    shift-right: [w71] -> w52
    shift-left: w45 -> [w72]
    tunnel: w43 -> [w70]
    stop <- w75 stop-if-true
    n57 = event shown="[7] \"Output mode LS335\": Value Change" {
      selector: _ -> [_ _ _ _ _ _ _ _]
      dyn-events: _ -> [_ _ _ _ _ _ _ _]
      timeout: _ -> [_ _ _ _ _ _ _ _]
      tunnel: [_ w78 TRUE ("Discard?") TRUE ("Discard?") _ _ _ _] -> w75
      tunnel: w74 -> [w76 w77 w79 w140 w144 w150 w157 w169]
      tunnel: [w76 w77 w79 w88 w144 w150 w157 w169] -> w73
      tunnel: w72 -> [_ _ _ w124 w146 w153 w155 w167]
      tunnel: [_ _ _ w124 w145 w151 w154 w166] -> w71
      tunnel: w70 -> [_ _ _ _ _ w152 _ _]
      event Timeout {
        n58 = event-data() -> ()  [unwired: 1 in, 1 out]
      }
      event Panel Close? {
        w78 = TRUE ("Discard?")
        n59 = event-data() -> ()  [unwired: 1 in, 1 out]
        n60 = event-data("Discard?"=w78) -> ()  [unwired: 1 in, 1 out]
      }
      event "Cancel": Value Change {
        n61 = event-data() -> ()  [unwired: 1 in, 1 out]
      }
      event "Apply All": Value Change {
        w119 = FALSE ("Defaults.DLTS properties.Pulse 2")
        n62 = event-data() -> ()  [unwired: 1 in, 1 out]
        n63 = Unbundle By Name("PID") -> ("Gain (P)"=w83:dbl, "Reset (I)"=w82:dbl, "Rate (D)"=w81:u16)
        n64 = Cast Unit Bases(0:"Stabilization rate") -> (2:w133:dbl)  [unwired: 1 in]
        n65 = Cast Unit Bases(0:"Stabilization delta") -> (2:w132:dbl)  [unwired: 1 in]
        n66 = Bundle By Name(cluster=w140, "MFIA.Address"="Address", "MFIA.Use compensation"="Use user compensation", "MFIA.Shut down gracefully"="Safely shutdown on exit", "Temp ctrl.Lakeshore 325.VISA name"="VISA name LS325", "Temp ctrl.Gain (P)"=w83, "Temp ctrl.Reset (I)"=w82, "Temp ctrl.Rate (D)"=w81, "Temp ctrl.Lakeshore 325.Loop"="Loop  LS325", "Temp ctrl.Lakeshore 325.Heater Range"="Heater range LS325", "Temp ctrl.Lakeshore 325.Heater Resistance"="Heater resistance LS325", "Temp ctrl.Lakeshore 325.Sample sensor"="Sample sensor LS325", "Temp ctrl.Lakeshore 325.Fast sensor"="Fast sensor LS325", "Temp ctrl.Lakeshore 325.Slow sensor"="Slow sensor LS325", "Temp ctrl.Stabilization rate"=w133, "Temp ctrl.Stabilization delta"=w132, "Temp ctrl.Type"="Temp type", "Temp ctrl.Custom temp ctrl"="Custom temp ctrl", "Other.Enable OriginLab"=FALSE, "Other.Reader mode"="Reader mode", "Source-meter.Type"="Source-meter type", "Source-meter.Custom source-meter"="Custom source-meter", "Source-meter.Keithley 2600.VISA name"="VISA name Keithley 2600") -> (w123:T11)
        n67 = Bundle("VISA name LS335"="VISA name LS335", "Loop  LS335"="Loop  LS335", "Sample sensor LS335"="Sample sensor LS335", "Fast sensor LS335"="Fast sensor LS335", "Slow sensor LS335"="Slow sensor LS335", "Heater range LS335"="Heater range LS335", "Heater output LS335"="Heater output LS335", "Output mode LS335"="Output mode LS335") -> (w96:T20)  [unwired: 1 in]
        n68 = Bundle("VISA name LS332"="VISA name LS332", "Loop  LS332"="Loop  LS332", "Heater range LS332"="Heater range LS332", "Sample sensor LS332"="Sample sensor LS332", "Fast sensor LS332"="Fast sensor LS332", "Slow sensor LS332"="Slow sensor LS332") -> (w97:T21)  [unwired: 1 in]
        n69 = Bundle("VISA name LS331"="VISA name LS331", "Loop  LS331"="Loop  LS331", "Heater range LS331"="Heater range LS331", "Sample sensor LS331"="Sample sensor LS331", "Fast sensor LS331"="Fast sensor LS331", "Slow sensor LS331"="Slow sensor LS331") -> (w98:T22)  [unwired: 1 in]
        n70 = Bundle By Name(cluster=w123, "Defaults.DLTS properties.Pulse 2"=w119, "Defaults.LDLTS properties.Pulse 2"=w119, "Other.Auto-save"="Auto-save", "Temp ctrl.Lakeshore 331"=w98, "Temp ctrl.Lakeshore 332"=w97, "Temp ctrl.Lakeshore 335"=w96) -> (w89:T11)
        n71 = Bundle By Name(cluster=w89, "Defaults.IV properties"="IV properties", "Defaults.CV properties"="CV properties", "Defaults.DLTS properties"="DLTS properties", "Defaults.LDLTS properties"="LDLTS properties") -> (w88:T11)
      }
      event "Refresh": Value Change {
        n72 = event-data() -> ()  [unwired: 1 in, 1 out]
        n73 = call <instrlib>:"ziLVInit.vi"("Error In"=w146) -> ("Error Out"=w147:errorcluster, "ziHandle"=w148:T23)  [unwired: 9 in]
        n74 = call <instrlib>:"ziDiscoveryListDevices.vi"("Error In"=w147, "ziHandle In"=w148) -> ("Error Out"=w142:errorcluster, "DevicesList"=w141:string[], "ziHandle Out"=w149:T23)  [unwired: 7 in]
        n75 = property on="Address" class="CmbBox"(error in=w142, "Strings[]"=w141) -> (error out=w143:errorcluster)  [unwired: 1 in, 1 out]
        n76 = call <instrlib>:"ziClose.vi"("Error In"=w143, "Handle In"=w149) -> ("Error Out"=w145:errorcluster)  [unwired: 2 in, 1 out]
      }
      event "Help": Value Change {
        n77 = event-data() -> ()  [unwired: 1 in, 6 out]
        n78 = call "OpenDoc Browser.vi"("error in (no error)"=w153, "File"=w152) -> ("error out"=w151:errorcluster)  [unwired: 9 in]
      }
      event "Temp type": Value Change {
        n79 = event-data() -> ("NewVal"=w158:T2)  [unwired: 1 in]
        n80 = case shown="\"Lake Shore 335\"" w158 {
          tunnel: [T19."Enabled" ("Disabled") w161] -> w156
          frame "Custom", Default {
          }
          frame "Lake Shore 335" {
            n81 = local read "Output mode LS335"() -> (w160:T4)
            n82 = case shown="\"Off\", Default" w160 {
              tunnel: [T19."Disabled and Grayed Out" ("Disabled") T19."Enabled" ("Disabled")] -> w161
              frame "Off", Default {
              }
              frame "Closed Loop PID" {
              }
            }
          }
        }
        n83 = property on="PID" class="Clust (strict)"(error in=w155, "DisabledEnum"=w156) -> (error out=w154:errorcluster)  [unwired: 1 in, 1 out]
      }
      event "Output mode LS335": Value Change {
        n84 = event-data() -> ("NewVal"=w165:T4)  [unwired: 1 in]
        n85 = local read "Temp type"() -> (w164:T2)
        n86 = case shown="\"Lake Shore 335\"" w164 {
          tunnel: [T19."Enabled" ("Disabled") w172] -> w168
          tunnel: w165 -> [_ w171]
          frame "Custom", Default {
          }
          frame "Lake Shore 335" {
            n87 = case shown="\"Off\", Default" w171 {
              tunnel: [T19."Disabled and Grayed Out" ("Disabled") T19."Enabled" ("Disabled")] -> w172
              frame "Off", Default {
              }
              frame "Closed Loop PID" {
              }
            }
          }
        }
        n88 = property on="PID" class="Clust (strict)"(error in=w167, "DisabledEnum"=w168) -> (error out=w166:errorcluster)  [unwired: 1 in, 1 out]
      }
    }
  }
  "Settings" <- w51
  "Error Out" <- w52
